vi "Record Live Video.vi"() -> ()   [LabVIEW 2015]
panel:
  in  "FileNmae":string="Eye Video"
  in  "LogDir":path=path "d:/"
  out "error out":errorcluster
  in  "Stop (F)":bool
  out "Image Out":T1(plugin-control)
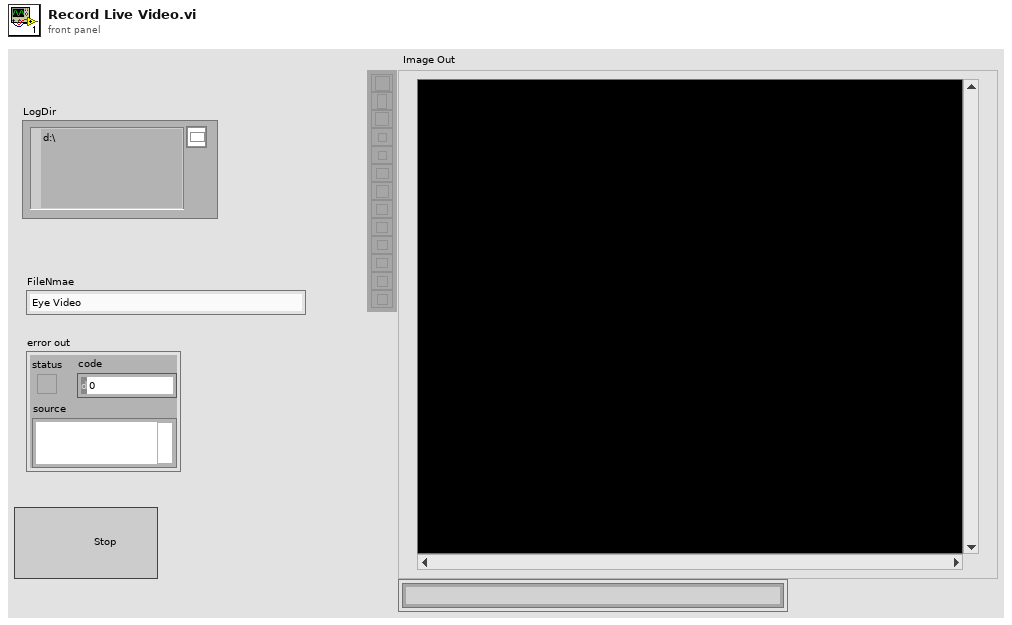
[diagram p1: front panel]
types:
  T1 = typedef "IMAQ Image.ctl" = refnum<image>
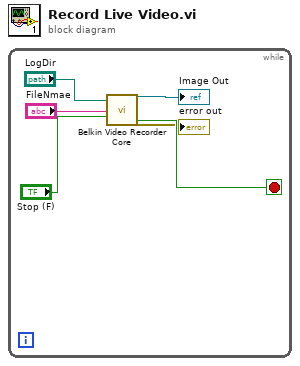
[diagram p0: block diagram]
diagram:
  n1 = while {
    stop <- w4 stop-if-true
    n2 = call "Belkin Video Recorder Core.vi"("LogDir"="LogDir", "FileNmae"="FileNmae", "Stop (F)"="Stop (F)") -> ("Image Out"=→"Image Out":T1, "Stopped"=w4:bool, "error out"=→"error out":errorcluster)  [unwired: 21 in, 1 out]
  }
